vi "Panel.vi"() -> ()   [LabVIEW 2020]
uses:
  <vilib>/measure/NI_MABase.lvlib
panel:
  out "Numeric 3":dbl
  out "Numeric 2":i32
  out "Numeric":i32
  out "Cursor 1(YL)":T1={"State"=1.1157556270096463, "EDEG"=1.1157556270096463, "Time"=1.1157556270096463, "Gauge"=0.0}
  out "Cursor 2(BL)":T1={"State"=1.1157556270096463, "EDEG"=1.1157556270096463, "Time"=1.1157556270096463, "Gauge"=0.0}
  out "Total Samples":dbl
  in  "Trigger Treshold(V)":dbl
  in  "Sample Rate(Hz)":dbl
  in  "Capture Period(Sec)":dbl
  out "Commutation":waveform(i32)(graph)={"t0"=timestamp(0 s since 1904-01-01), "dt"=0.001, "Y"=[1, 1, 1, 1, 1, 1, 1, 1, 1, 1, 1, 1, 1, 1, 1, 1, 6, 6, 6, 6, 6, 6, 6, 6, 6, 6, 6, 6, 6, 6, 6, 6, 6, 5, 5, 5, 5, 5, 5, 5, 5, 5, 5, 5, 5, 5, 5, 5, 5, 5, 4, 4, 4, 4, 4, 4, 4, 4, 4, 4, 4, 4, 4, 4, 4, 4, 3, 3, 3, 3, 3, 3, 3, 3, 3, 3, 3, 3, 3, 3, 3, 3, 3, 2, 2, 2, 2, 2, 2, 2, 2, 2, 2, 2, 2, 2, 2, 2, 2, 2, 1, 1, 1, 1, 1, 1, 1, 1, 1, 1, 1, 1, 1, 1, 1, 1, 6, 6, 6, 6, 6, 6, 6, 6, 6, 6, 6, 6, 6, 6, 6, 6, 6, 5, 5, 5, 5, 5, 5, 5, 5, 5, 5, 5, 5, 5, 5, 5, 5, 5, 4, 4, 4, 4, 4, 4, 4, 4, 4, 4, 4, 4, 4, 4, 4, 4, 3, 3, 3, 3, 3, 3, 3, 3, 3, 3, 3, 3, 3, 3, 3, 3, 3, 2, 2, 2, 2, 2, 2, 2, 2, 2, 2, 2, 2, 2, 2, 2, 2, 2, 1, 1, 1, 1, 1, 1, 1, 1, 1, 1, 1, 1, 1, 1, 1, 1, 6, 6, 6, 6, 6, 6, 6, 6, 6, 6, 6, 6, 6, 6, 6, 6, 6, 5, 5, 5, 5, 5, 5, 5, 5, 5, 5, 5, 5, 5, 5, 5, 5, 5, 4, 4, 4, 4, 4, 4, 4, 4, 4, 4, 4, 4, 4, 4, 4, 4, 3, 3, 3, 3, 3, 3, 3, 3, 3, 3, 3, 3, 3, 3, 3, 3, 3, 2, 2, 2, 2, 2, 2, 2, 2, 2, 2, 2, 2, 2, 2, 2, 2, 2, 1, 1, 1, 1, 1, 1, 1, 1, 1, 1, 1, 1, 1, 1, 1, 1, 6, 6, 6, 6, 6, 6, 6, 6, 6, 6, 6, 6, 6, 6, 6, 6, 6, 5, 5, 5, 5, 5, 5, 5, 5, 5, 5, 5, 5, 5, 5, 5, 5, 5, 4, 4, 4, 4, 4, 4, 4, 4, 4, 4, 4, 4, 4, 4, 4, 4, 3, 3, 3, 3, 3, 3, 3, 3, 3, 3, 3, 3, 3, 3, 3, 3, 3, 2, 2, 2, 2, 2, 2, 2, 2, 2, 2, 2, 2, 2, 2, 2, 2, 2, 1, 1, 1, 1, 1, 1, 1, 1, 1, 1, 1, 1, 1, 1, 1, 1, 6, 6, 6, 6, 6, 6, 6, 6, 6, 6, 6, 6, 6, 6, 6, 6, 6, 5, 5, 5, 5, 5, 5, 5, 5, 5, 5, 5, 5, 5, 5, 5, 5, 5, 4, 4, 4, 4, 4, 4, 4, 4, 4, 4, 4, 4, 4, 4, 4, 4, 3, 3, 3, 3, 3, 3, 3, 3, 3, 3, 3, 3, 3, 3, 3, 3, 3, 2, 2, 2, 2, 2, 2, 2, 2, 2, 2, 2, 2, 2, 2, 2, 2, 2, 1, 1, 1, 1, 1, 1, 1, 1, 1, 1, 1, 1, 1, 1, 1, 1, 6, 6, 6, 6, 6, 6, 6, 6, 6, 6, 6, 6, 6, 6, 6, 6, 6, 5, 5, 5, 5, 5, 5, 5, 5, 5, 5, 5, 5, 5, 5, 5, 5, 5, 4, 4, 4, 4, 4, 4, 4, 4, 4, 4, 4, 4, 4, 4, 4, 4, 3, 3, 3, 3, 3, 3, 3, 3, 3, 3, 3, 3, 3, 3, 3, 3, 3, 2, 2, 2, 2, 2, 2, 2, 2, 2, 2, 2, 2, 2, 2, 2, 2, 2, 1, 1, 1, 1, 1, 1, 1, 1, 1, 1, 1, 1, 1, 1, 1, 1, 6, 6, 6, 6, 6, 6, 6, 6, 6, 6, 6, 6, 6, 6, 6, 6, 6, 5, 5, 5, 5, 5, 5, 5, 5, 5, 5, 5, 5, 5, 5, 5, 5, 5, 4, 4, 4, 4, 4, 4, 4, 4, 4, 4, 4, 4, 4, 4, 4, 4, 3, 3, 3, 3, 3, 3, 3, 3, 3, 3, 3, 3, 3, 3, 3, 3, 3, 2, 2, 2, 2, 2, 2, 2, 2, 2, 2, 2, 2, 2, 2, 2, 2, 2, 1, 1, 1, 1, 1, 1, 1, 1, 1, 1, 1, 1, 1, 1, 1, 1, 6, 6, 6, 6, 6, 6, 6, 6, 6, 6, 6, 6, 6, 6, 6, 6, 6, 5, 5, 5, 5, 5, 5, 5, 5, 5, 5, 5, 5, 5, 5, 5, 5, 5, 4, 4, 4, 4, 4, 4, 4, 4, 4, 4, 4, 4, 4, 4, 4, 4, 3, 3, 3, 3, 3, 3, 3, 3, 3, 3, 3, 3, 3, 3, 3, 3, 3, 2, 2, 2, 2, 2, 2, 2, 2, 2, 2, 2, 2, 2, 2, 2, 2, 2, 1, 1, 1, 1, 1, 1, 1, 1, 1, 1, 1, 1, 1, 1, 1, 1, 6, 6, 6, 6, 6, 6, 6, 6, 6, 6, 6, 6, 6, 6, 6, 6, 6, 5, 5, 5, 5, 5, 5, 5, 5, 5, 5, 5, 5, 5, 5, 5, 5, 5, 4, 4, 4, 4, 4, 4, 4, 4, 4, 4, 4, 4, 4, 4, 4, 4, 3, 3, 3, 3, 3, 3, 3, 3, 3, 3, 3, 3, 3, 3, 3, 3, 3, 2, 2, 2, 2, 2, 2, 2, 2, 2, 2, 2, 2, 2, 2, 2, 2, 2, 1, 1, 1, 1, 1, 1, 1, 1, 1, 1, 1, 1, 1, 1, 1, 1, 6, 6, 6, 6, 6, 6, 6, 6, 6, 6, 6, 6, 6, 6, 6, 6, 6, 5, 5, 5, 5, 5, 5, 5, 5, 5, 5, 5, 5, 5, 5, 5, 5, 5, 4, 4, 4, 4, 4, 4, 4, 4, 4, 4, 4, 4, 4, 4, 4, 4, 3, 3, 3, 3, 3, 3, 3, 3, 3, 3, 3, 3, 3, 3, 3, 3, 3, 2, 2, 2, 2, 2, 2, 2, 2, 2, 2, 2, 2, 2, 2, 2, 2, 2]}
  out "Hall Effect Outputs":dynamicdata(graph)=[{"t0"=timestamp(0 s since 1904-01-01), "dt"=0.001, "Y"=array[1000 elements]}, {"t0"=timestamp(0 s since 1904-01-01), "dt"=0.001, "Y"=array[1000 elements]}, {"t0"=timestamp(0 s since 1904-01-01), "dt"=0.001, "Y"=array[1000 elements]}]
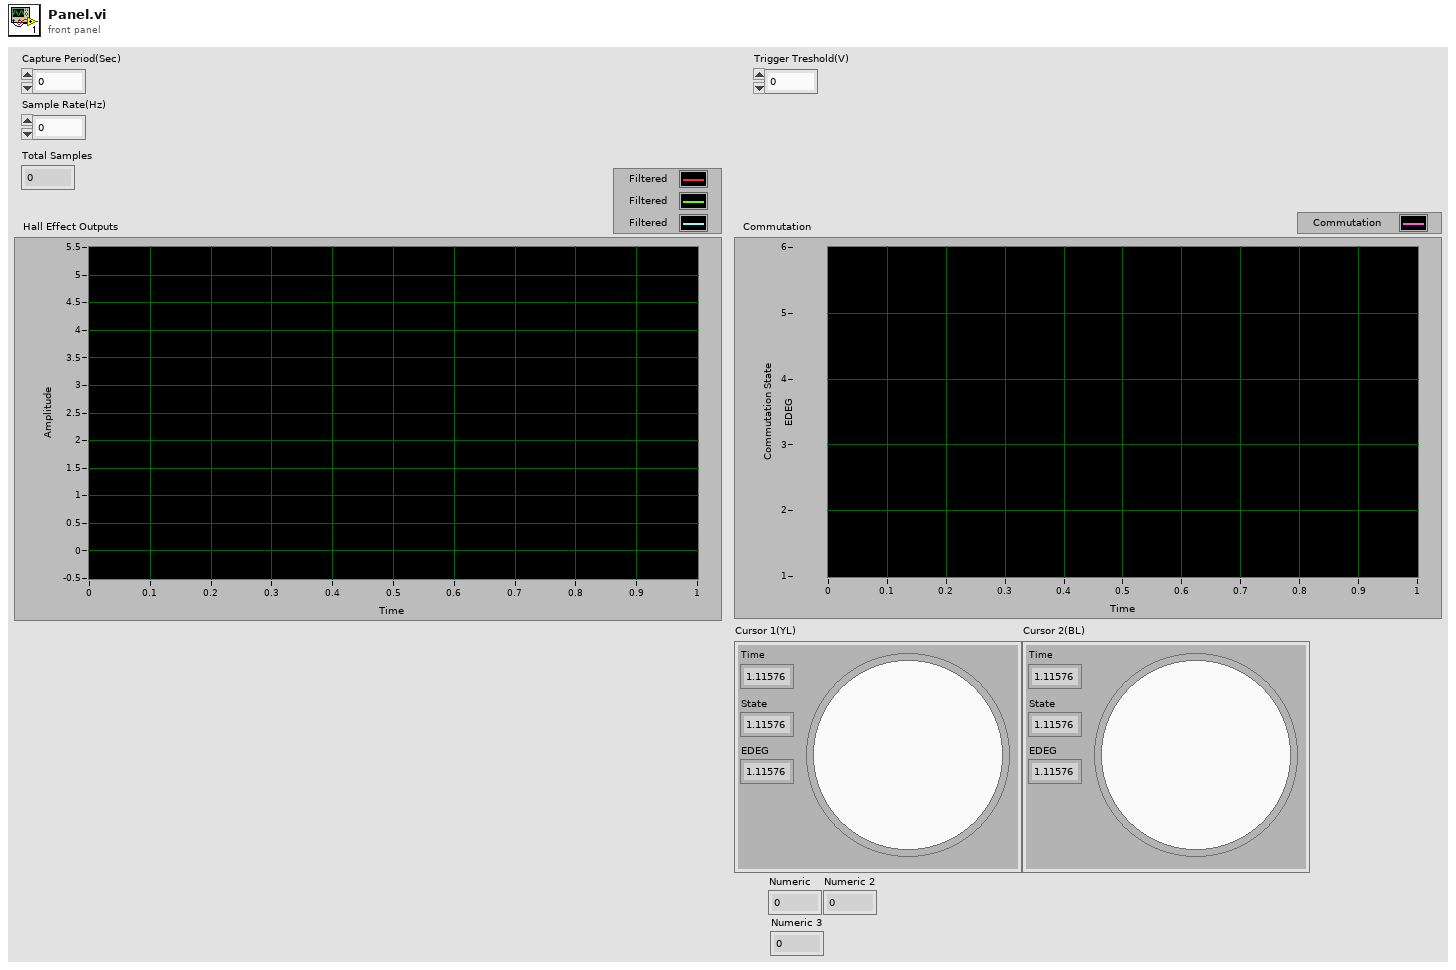
[diagram p1: front panel]
types:
  T1 = cluster{"State":dbl, "EDEG":dbl, "Time":dbl, "Gauge":dbl}
  T2 = cluster{"frequency":dbl, "amplitude":dbl, "phase":dbl}[]
  T3 = cluster{"Name":string, "Color":u32, "Style":u8, "Point Style":u8, "Name Visible":bool, "Allow Drag":bool, "Annotation Mode":u32, "Plot":i32, "Index":i32, "Position":cluster{"X":dbl, "Y":dbl}, "X Scale":u32, "Y Scale":u32, "Show Arrow":bool, "Lock Name":bool, "Plot Area":i32, "Label Offset":cluster{"X":i32, "Y":i32}}
  T4 = cluster{"Name":string, "Color":u32, "Style":u8, "Point Style":u8, "Name Visible":bool, "Allow Drag":bool, "Annotation Mode":u32, "Plot":i32, "Index":i32, "Position":cluster{"X":dbl, "Y":dbl}, "X Scale":u32, "Y Scale":u32, "Show Arrow":bool, "Lock Name":bool, "Plot Area":i32, "Label Offset":cluster{"X":i32, "Y":i32}}[]
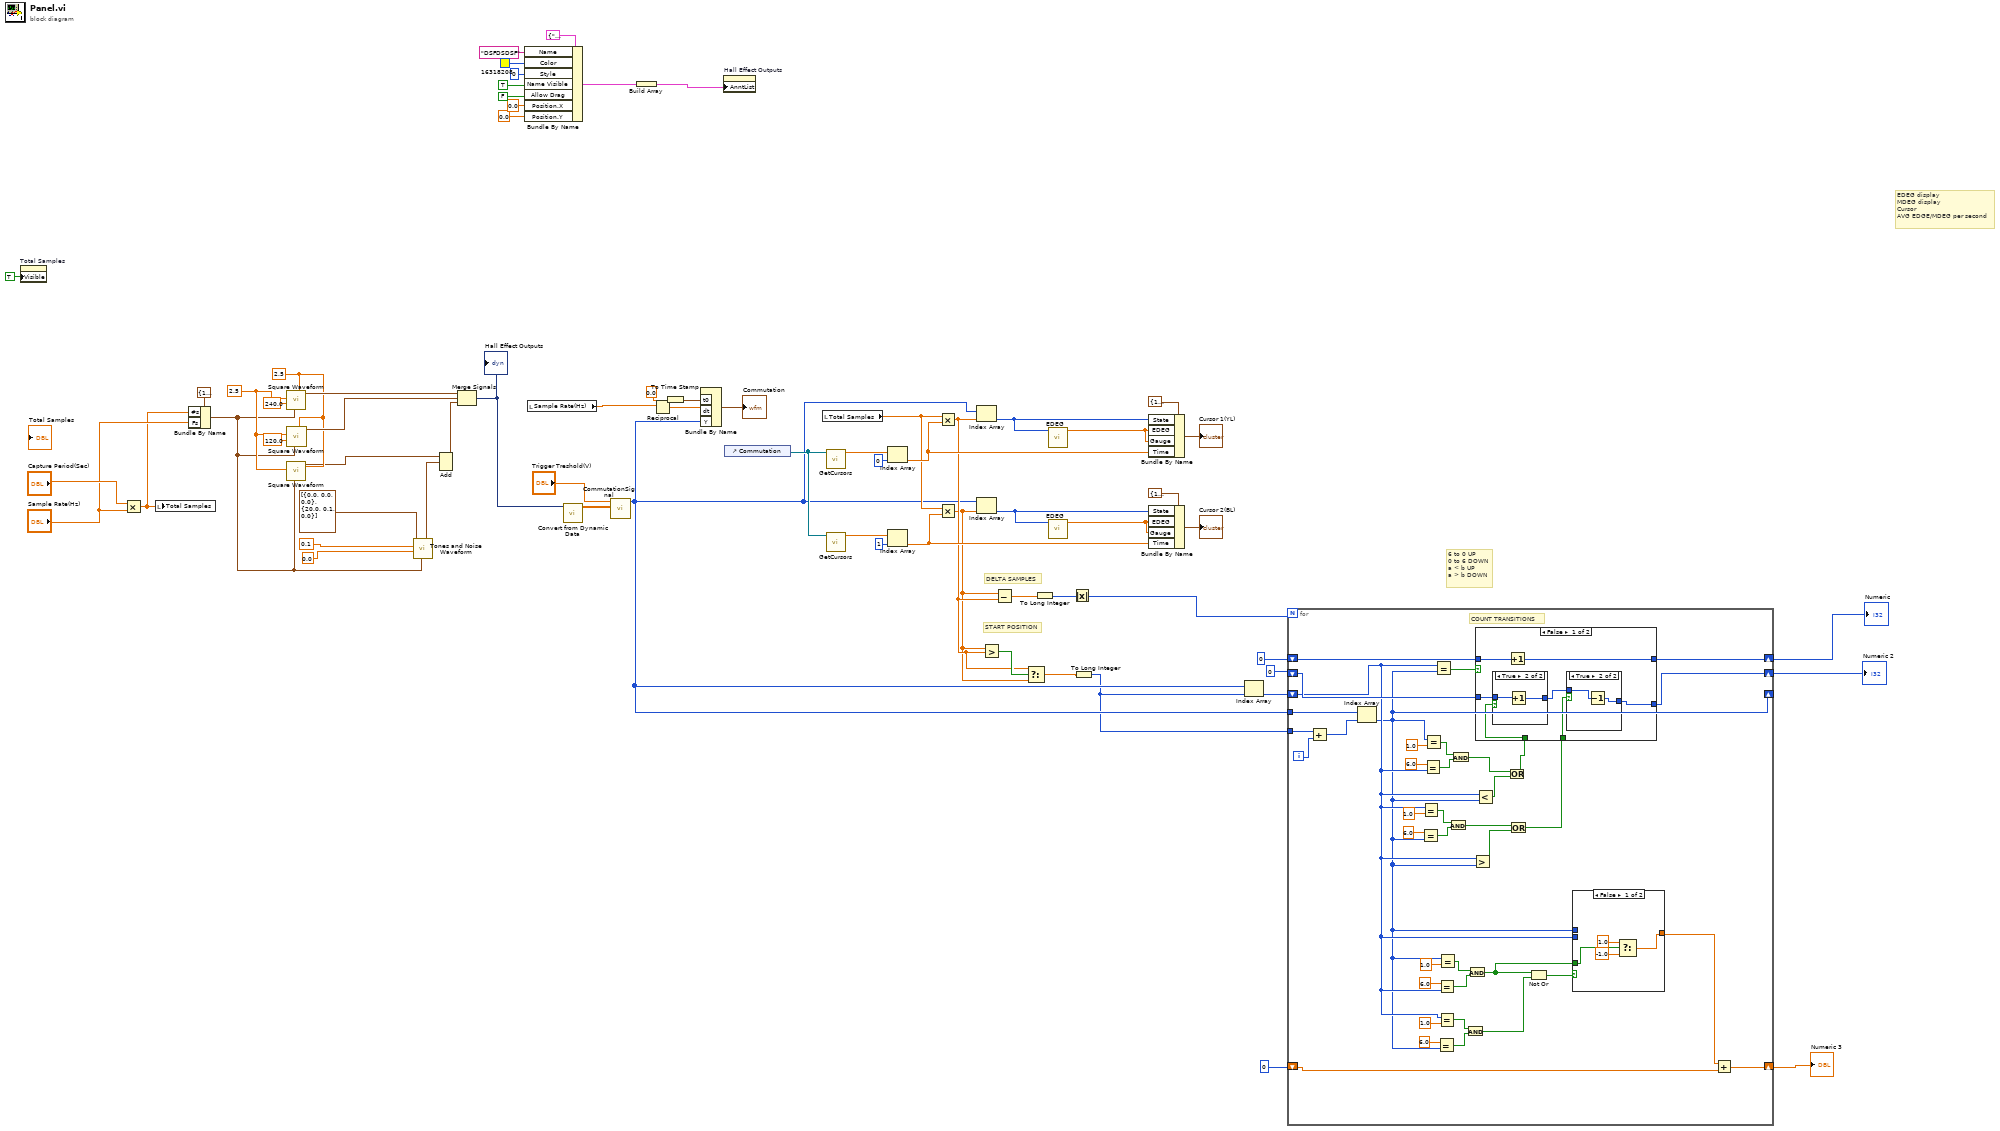
[diagram p0: block diagram]
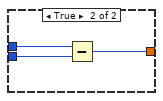
[diagram p2: hidden frame]
diagram:
  w63 = 2.5 ("offset")
  w64 = 2.5 ("amplitude")
  # "6 to 0 UP\n0 to 6 DOWN\na < b UP\na > b DOWN"
  # "START POSITION"
  # "DELTA SAMPLES"
  # "EDEG display\nMDEG display\nCursor\nAVG EDGE/MDEG per second"
  n1 = property on="Total Samples" class="DigNum (strict)"("Visible"=TRUE) -> ()  [unwired: 2 in, 2 out]
  n2 = Multiply(x="Capture Period(Sec)", y="Sample Rate(Hz)") -> (x*y=w22:dbl)
  n3 = local write "Total Samples"(w22) -> ()
  n4 = Bundle By Name(cluster=cluster{"Fs":dbl, "#s":dbl} {"Fs"=1000.0, "#s"=1000.0} ("sampling info"), "#s"=w22, "Fs"="Sample Rate(Hz)") -> (w20:cluster{"Fs":dbl, "#s":dbl})
  n5 = call <vilib>:"Square Waveform.vi"("offset"=w63, "sampling info"=w20, "phase"=240.0, "amplitude"=w64) -> ("signal out"=w66:waveform(dbl))  [unwired: 6 in, 1 out]
  n6 = call <vilib>:"Square Waveform.vi"("offset"=w63, "sampling info"=w20, "amplitude"=w64) -> ("signal out"=w49:waveform(dbl))  [unwired: 7 in, 1 out]
  n7 = call <vilib>:"Square Waveform.vi"("offset"=w63, "sampling info"=w20, "phase"=120.0, "amplitude"=w64) -> ("signal out"=w65:waveform(dbl))  [unwired: 6 in, 1 out]
  n8 = call <vilib>:"Tones and Noise Waveform.vi"("sampling info"=w20, "offset"=0.0, "noise (rms)"=0.1, "tones"=T2 [{"frequency"=0.0, "amplitude"=0.0, "phase"=0.0}, {"frequency"=20.0, "amplitude"=0.1, "phase"=0.0}]) -> ("signal out"=w48:waveform(dbl))  [unwired: 6 in, 1 out]
  n9 = Add(1:w48, 2:w49) -> (0:w47:waveform(dbl))  [unwired: 1 in, 1 out]
  n10 = Merge Signals(w66, w65, w47) -> (w21:dynamicdata)
  "Hall Effect Outputs" <- w21
  n11 = Bundle By Name(cluster=T3 {"Name"="", "Color"=0, "Style"=0, "Point Style"=0, "Name Visible"=FALSE, "Allow Drag"=FALSE, "Annotation Mode"=0, "Plot"=0, "Index"=0, "Position"={"X"=0.0, "Y"=0.0}, "X Scale"=0, "Y Scale"=0, "Show Arrow"=FALSE, "Lock Name"=FALSE, "Plot Area"=0, "Label Offset"={"X"=1, "Y"=1}}, "Name"="DSFDSDSF", "Color"=u32 16318208, "Style"=u8 0, "Name Visible"=TRUE, "Allow Drag"=FALSE, "Position.X"=0.0, "Position.Y"=0.0) -> (w54:T3)
  n12 = local read "Sample Rate(Hz)"() -> (w19:dbl)
  n13 = call "Convert from Dynamic Data"("Dynamic Data Type"=w21) -> ("Array"=w25:dbl[][])  [unwired: 3 in]
  n14 = call "CommutationSignal.vi"("Array in"=w25, "Treshold"="Trigger Treshold(V)") -> ("Array out"=w9:i32[])  [unwired: 9 in]
  n15 = Build Array(w54) -> (w53:T4)
  n16 = Reciprocal(x=w19) -> (1/x=w38:dbl)
  n17 = To Time Stamp(1:0.0) -> (0:w46:timestamp)
  n18 = Bundle By Name("t0"=w46, "dt"=w38, "Y"=w9) -> (→"Commutation":waveform(i32))  [unwired: 1 in]
  n19 = property on="Hall Effect Outputs" class="WFGraph (strict)"("AnntList"=w53) -> ()  [unwired: 2 in, 2 out]
  n20 = control-ref of="Commutation"() -> (w27:refnum<vi>)
  n21 = local read "Total Samples"() -> (w26:dbl)
  n22 = call "GetCursors.vi"("WaveformGraph in"=w27) -> ("Cursor Positions"=w40:dbl[])  [unwired: 10 in]
  n23 = call "GetCursors.vi"("WaveformGraph in"=w27) -> ("Cursor Positions"=w34:dbl[])  [unwired: 10 in]
  n24 = Index Array(array=w40, index=0) -> (element=w36:dbl)
  n25 = Index Array(array=w34, index=1) -> (element=w31:dbl)
  n26 = Multiply(x=w26, y=w36) -> (x*y=w14:dbl)
  n27 = Multiply(x=w26, y=w31) -> (x*y=w13:dbl)
  n28 = Index Array(array=w9, index=w14) -> (element=w41:i32)
  n29 = Index Array(array=w9, index=w13) -> (element=w12:i32)
  n30 = Greater?(x=w13, y=w14) -> (0:w15:bool)
  n31 = Subtract(x=w13, y=w14) -> (x-y=w17:dbl)
  n32 = Select(t=w14, s=w15, f=w13) -> (s? t:f=w7:dbl)
  n33 = To Long Integer(number=w17) -> (32bit integer=w16:i32)
  n34 = call "EDEG.vi"("State"=w41) -> ("EDEG"=w35:dbl)  [unwired: 10 in]
  n35 = call "EDEG.vi"("State"=w12) -> ("EDEG"=w30:dbl)  [unwired: 10 in]
  n36 = Absolute Value(x=w16) -> (abs(x)=w5:i32)
  n37 = To Long Integer(number=w7) -> (32bit integer=w6:i32)
  n38 = Bundle By Name(cluster=T1 {"State"=1.1157556270096463, "EDEG"=1.1157556270096463, "Time"=1.1157556270096463, "Gauge"=30.288084445625785} ("Cursor 2(BL)"), "State"=w41, "EDEG"=w35, "Gauge"=w35, "Time"=w36) -> (→"Cursor 1(YL)":T1)
  n39 = Bundle By Name(cluster=T1 {"State"=1.1157556270096463, "EDEG"=1.1157556270096463, "Time"=1.1157556270096463, "Gauge"=30.288084445625785} ("Cursor 2(BL)"), "State"=w12, "EDEG"=w30, "Gauge"=w30, "Time"=w31) -> (→"Cursor 2(BL)":T1)
  n40 = Index Array(array=w9, index=w6) -> (element=w10:i32)
  n41 = for {
    N: w5 -> [_]
    shift-right: [w105] -> w8
    shift-left: 0 -> [w107]
    tunnel: w9 -> [w106]
    shift-right: [w79] -> _
    shift-left: w10 -> [w80]
    tunnel: w6 -> [w102]
    shift-right: [w85] -> w3
    shift-left: 0 -> [w86]
    shift-right: [w69] -> w1
    shift-left: 0 -> [w70]
    i -> [w104]
    # "COUNT TRANSITIONS"
    n42 = Add(x=w102, y=w104) -> (x+y=w103:i32)
    n43 = Index Array(array=w106, index=w103) -> (element=w79:i32)
    n44 = Equal?(x=6.0, y=w79) -> (x = y?=w95:bool)
    n45 = Equal?(x=w80, y=1.0) -> (x = y?=w96:bool)
    n46 = Equal?(x=6.0, y=w80) -> (x = y?=w99:bool)
    n47 = Equal?(x=w79, y=1.0) -> (x = y?=w100:bool)
    n48 = Equal?(x=w80, y=w79) -> (x = y?=w101:bool)
    n49 = Equal?(x=6.0, y=w79) -> (x = y?=w75:bool)
    n50 = Equal?(x=6.0, y=w80) -> (x = y?=w77:bool)
    n51 = Equal?(x=w80, y=1.0) -> (x = y?=w76:bool)
    n52 = Equal?(x=w79, y=1.0) -> (x = y?=w78:bool)
    n53 = And(x=w96, y=w95) -> (x .and. y?=w92:bool)
    n54 = And(x=w100, y=w99) -> (x .and. y?=w90:bool)
    n55 = And(x=w76, y=w75) -> (x .and. y?=w74:bool)
    n56 = And(x=w78, y=w77) -> (x .and. y?=w72:bool)
    n57 = Greater?(x=w80, y=w79) -> (0:w91:bool)
    n58 = Less?(x=w80, y=w79) -> (x < y?=w89:bool)
    n59 = Or(x=w90, y=w89) -> (x .or. y?=w88:bool)
    n60 = Or(x=w92, y=w91) -> (x .or. y?=w87:bool)
    n61 = case shown="False" w101 {
      tunnel: w107 -> [w121 w129]
      tunnel: [w120 w129] -> w105
      tunnel: w88 -> [w119 _]
      tunnel: w87 -> [w118 _]
      tunnel: w86 -> [w117 w128]
      tunnel: [w115 w128] -> w85
      frame False {
        n62 = case shown="True" w119 {
          tunnel: w117 -> [w125 w127]
          tunnel: [w125 w126] -> w116
          frame False {
          }
          frame True {
            n63 = Increment(x=w127) -> (x+1=w126:i32)
          }
        }
        n64 = Increment(x=w121) -> (x+1=w120:i32)
        n65 = case shown="True" w118 {
          tunnel: w116 -> [w122 w124]
          tunnel: [w122 w123] -> w115
          frame False {
          }
          frame True {
            n66 = Decrement(x=w124) -> (x-1=w123:i32)
          }
        }
      }
      frame True {
      }
    }
    n67 = Not Or(1:w74, 2:w72) -> (0:w73:bool)
    n68 = case shown="False" w73 {
      tunnel: w79 -> [_ w114]
      tunnel: w80 -> [_ w113]
      tunnel: [w108 w112] -> w71
      tunnel: w72 -> [w111 _]
      frame False {
        n69 = Select(t=1.0, s=w111, f=-1.0) -> (s? t:f=w108:dbl)
      }
      frame True {
        n70 = Subtract(x=w114, y=w113) -> (x-y=w112:i32)
      }
    }
    n71 = Add(x=w71, y=w70) -> (x+y=w69:dbl)
  }
  "Numeric" <- w8
  "Numeric 2" <- w3
  "Numeric 3" <- w1
